vi "Close Data Logger.vi"(8 "error in":errorcluster, 11 "Log FIle Ref. In":refnum<file>) -> (0 "error out":errorcluster)   [LabVIEW 2024, in "dataLogger.lvlib"]
doc: "<b>Close Data Logger</b> API , close the open log file refnum ."
uses:
  dataLogger.lvlib
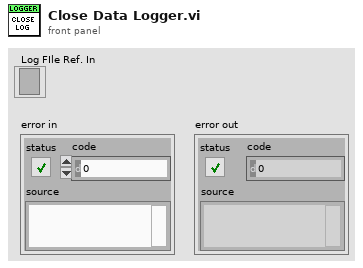
[diagram p1: front panel]
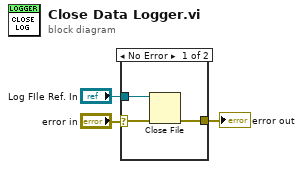
[diagram p0: block diagram]
diagram:
  n1 = case shown="No Error" "error in" {
    selector: "error in" -> [w6 w7]
    tunnel: [w5 w7] -> w2
    tunnel: "Log FIle Ref. In" -> [w4 _]
    frame No Error {
      n2 = Close File(refnum=w4, error in=w6) -> (error out=w5:errorcluster)  [unwired: 1 out]
    }
    frame Error {
    }
  }
  "error out" <- w2
